vi "Initialize.vi"(0 "Room Service Manager Model in":refnum<class "Room Service Manager Model.lvclass">, 11 "error in (no error)":errorcluster) -> (4 "Room Service Manager Model out":refnum<class "Room Service Manager Model.lvclass">, 15 "error out":errorcluster)   [LabVIEW 2023, in "Room Service Manager Model.lvlib" / "Room Service Manager Model.lvclass"]
uses:
  Room Service Manager Model.lvclass
  C:/Program Files/National Instruments/LabVIEW 2023/vi.lib/ActorFramework/Actor/Actor.lvclass
  Room Service Manager UI/Room Service Manager UI/Room Service Manager UI.lvclass
  Room Service Manager Model.lvclass/Room Service Manager Model.ctl
  <vilib>/ActorFramework/Actor/Actor.lvclass
  Room Service Manager Model Messages/Create Room Service Request Msg/Create Room Service Request Msg.lvclass
  C:/Users/bhaghyaraj/Trainings/NI Actor Framework/SDLC/Room Service Manager UI/Room Service Manager UI Messages/Create Room Service Request Msg/Create Room Service Request Msg.lvclass
  C:/Program Files/National Instruments/LabVIEW 2023/vi.lib/ActorFramework/Message/Message.lvclass
  C:/Users/bhaghyaraj/Trainings/NI Actor Framework/SDLC/Room Service Manager Model/Room Service Manager Model Messages/Create Room Service Request Msg/Create Room Service Request Msg.lvclass
  C:/Users/bhaghyaraj/Trainings/NI Actor Framework/SDLC/UI Base/UI Base/UI Base.lvclass
  C:/Users/bhaghyaraj/Trainings/NI Actor Framework/SDLC/Room Service Manager UI/Room Service Manager UI/Room Service Manager UI.lvclass
  C:/Users/bhaghyaraj/Trainings/NI Actor Framework/SDLC/Model Base/Model Base/Model Base.lvclass
  C:/Users/bhaghyaraj/Trainings/NI Actor Framework/SDLC/Interfaces/Model Base/Incoming Model Base Interface.lvclass
  C:/Users/bhaghyaraj/Trainings/NI Actor Framework/SDLC/Room Service Manager Model/Room Service Manager Model/Room Service Manager Model.lvclass
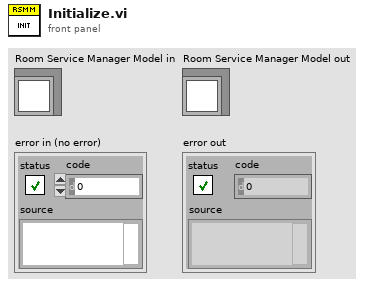
[diagram p1: front panel]
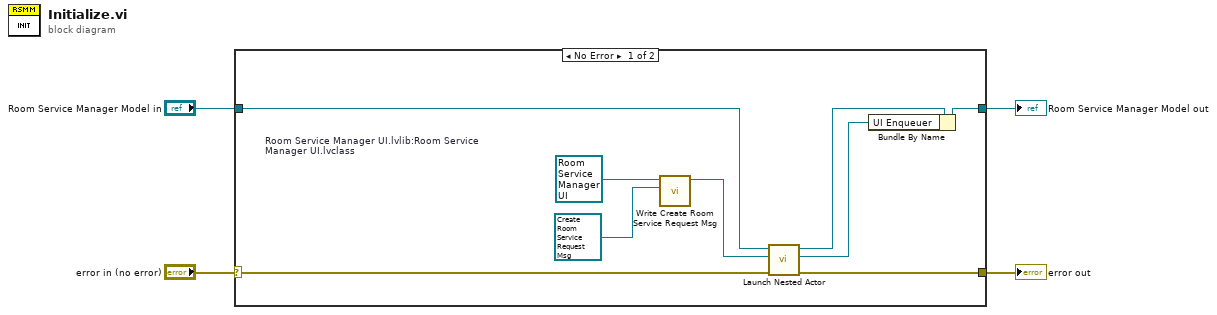
[diagram p0: block diagram]
diagram:
  n1 = case shown="No Error" "error in (no error)" {
    selector: "error in (no error)" -> [w8 w15]
    tunnel: [w13 w15] -> w1
    tunnel: [w10 w14] -> w2
    tunnel: "Room Service Manager Model in" -> [w12 w14]
    frame No Error {
      w7 = refnum<class "Room Service Manager UI.lvclass"> refnum  # Room Service Manager UI.lvlib:Room Service Manager UI.lvclass
      n2 = call "Write Create Room Service Request Msg.vi"("Room Service Manager UI.lvlib:Create Room Service Request Msg.lvclass"=refnum<class "Create Room Service Request Msg.lvclass"> refnum ("Room Service Manager Model.lvlib:Create Room Service Request Msg.lvclass"), "Room Service Manager UI in"=w7) -> ("Room Service Manager UI out"=w6:refnum<class "Room Service Manager UI.lvclass">)  [unwired: 9 in]
      n3 = call <vilib>:"Launch Nested Actor.vi"("error in (no error)"=w8, "Nested Actor"=w6, "Caller Actor in"=w12) -> ("error out"=w13:errorcluster, "Nested Actor's Enqueuer"=w9:refnum<class "Message Enqueuer.lvclass">, "Caller Actor out"=w11:refnum<class "Room Service Manager Model.lvclass">)  [unwired: 6 in]
      n4 = Bundle By Name(cluster=w11, "UI Enqueuer"=w9) -> (w10:refnum<class "Room Service Manager Model.lvclass">)
    }
    frame Error {
    }
  }
  "error out" <- w1
  "Room Service Manager Model out" <- w2
